vi "GeraSinalProximeter.vi"(0 "params":variant, 2 "Tx Aquisicao":dbl, 4 "estadoIn":variant) -> (15 "sinal":waveform(dbl), 18 "estadoOut":variant)   [LabVIEW 2017]
uses:
  Typedefs/Tipo_ParamsProximeter.ctl
  Typedefs/Tipo_ComponentesProximeter.ctl
  <vilib>/Analysis/NI_AALBase.lvlib
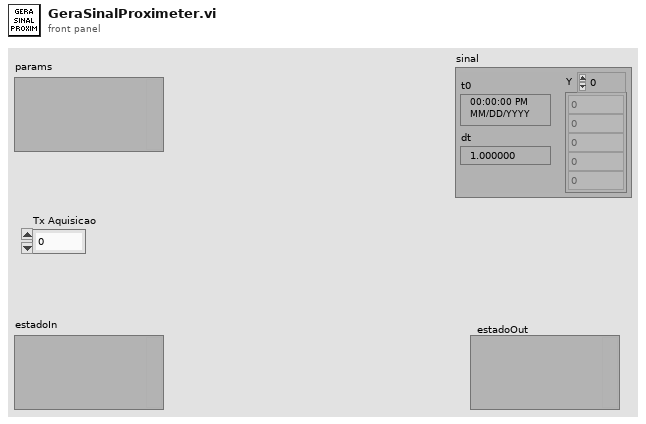
[diagram p1: front panel]
types:
  T1 = typedef "Tipo_ParamsProximeter.ctl" = cluster{"Rotacao":dbl, "Ruído":dbl, "Distância Eixo":dbl, "Fase":dbl, "Componentes":T2}
  T2 = typedef "Tipo_ComponentesProximeter.ctl" = cluster{"1xRPM":dbl, "2xRPM":dbl, "3xRPM":dbl, "4xRPM":dbl, "1/2xRPM":dbl, "1/3xRPM":dbl, "1/4xRPM":dbl, "0,45xRPM":dbl, "60Hz":dbl, "120Hz":dbl}
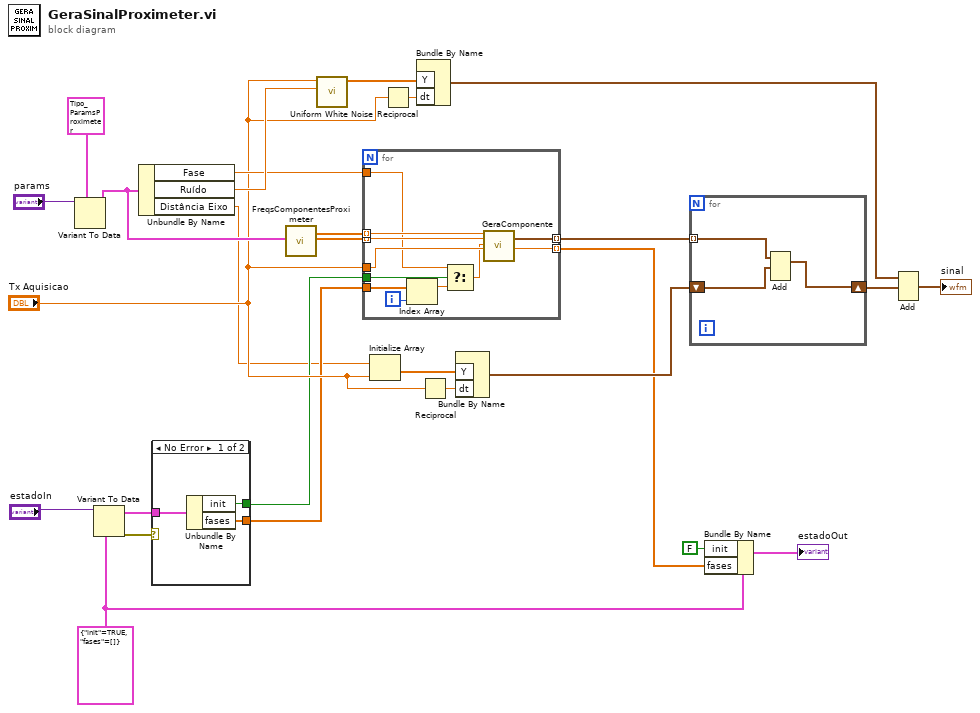
[diagram p0: block diagram]
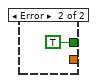
[diagram p2: hidden frame]
diagram:
  w22 = cluster{"init":bool, "fases":dbl[]} {"init"=TRUE, "fases"=[]}
  n1 = Variant To Data(type=T1 {"Rotacao"=0.0, "Ruído"=0.0, "Distância Eixo"=0.0, "Fase"=0.0, "Componentes"={"1xRPM"=0.0, "2xRPM"=0.0, "3xRPM"=0.0, "4xRPM"=0.0, "1/2xRPM"=0.0, "1/3xRPM"=0.0, "1/4xRPM"=0.0, "0,45xRPM"=0.0, "60Hz"=0.0, "120Hz"=0.0}} ("Tipo_ParamsProximeter"), Variant="params") -> (data=w10:T1)  [unwired: 1 in, 1 out]
  n2 = Variant To Data(type=w22, Variant="estadoIn") -> (data=w24:cluster{"init":bool, "fases":dbl[]}, error out=w23:errorcluster)  [unwired: 1 in]
  n3 = Unbundle By Name(w10) -> ("Fase"=w7:dbl, "Ruído"=w17:dbl, "Distância Eixo"=w1:dbl)
  n4 = case shown="No Error" w23 {
    tunnel: w24 -> [w30 _]
    tunnel: [w29 TRUE ("init")] -> w3
    tunnel: [w28 _] -> w4
    frame No Error {
      n5 = Unbundle By Name(w30) -> ("init"=w29:bool, "fases"=w28:dbl[])
    }
    frame Error {
    }
  }
  n6 = call "FreqsComponentesProximeter.vi"("Tipo_ParamsProximeter"=w10) -> ("AmplitComponentes"=w8:dbl[], "FreqsComponentes"=w9:dbl[])  [unwired: 17 in]
  n7 = call <vilib>:"Uniform White Noise.vi"("amplitude"=w17, "samples"="Tx Aquisicao") -> ("uniform white noise"=w16:dbl[])  [unwired: 8 in, 1 out]
  n8 = for {
    tunnel: w9 -> [w41] mode=indexing
    tunnel: w8 -> [w42] mode=indexing
    tunnel: w7 -> [w34]
    tunnel: "Tx Aquisicao" -> [w40]
    tunnel: [w39] -> w5 mode=indexing
    tunnel: w4 -> [w37]
    tunnel: w3 -> [w36]
    tunnel: [w32] -> w2 mode=indexing
    i -> [w38]
    n9 = Index Array(array=w37, index=w38) -> (element=w35:dbl)
    n10 = Select(t=w34, s=w36, f=w35) -> (s? t:f=w33:dbl)
    n11 = call "GeraComponente.vi"("Amplitude"=w42, "Frequencia"=w41, "Fase"=w33, "Tx Aquisicao"=w40) -> ("componente wfm"=w32:waveform(dbl), "fase saida"=w39:dbl)  [unwired: 14 in]
  }
  n12 = Initialize Array(w1, "Tx Aquisicao") -> (w13:dbl[])
  n13 = Reciprocal(x="Tx Aquisicao") -> (1/x=w15:dbl)
  n14 = Bundle By Name("Y"=w16, "dt"=w15) -> (w14:waveform(dbl))  [unwired: 1 in]
  n15 = Reciprocal(x="Tx Aquisicao") -> (1/x=w12:dbl)
  n16 = Bundle By Name("Y"=w13, "dt"=w12) -> (w11:waveform(dbl))  [unwired: 1 in]
  n17 = for {
    shift-right: [w44] -> w19
    shift-left: w11 -> [w45]
    tunnel: w2 -> [w43] mode=indexing
    n18 = Add(1:w45, 2:w43) -> (0:w44:waveform(dbl))  [unwired: 1 in, 1 out]
  }
  n19 = Bundle By Name(cluster=w22, "init"=FALSE, "fases"=w5) -> (→"estadoOut":cluster{"init":bool, "fases":dbl[]})
  n20 = Add(1:w19, 2:w14) -> (0:→"sinal":waveform(dbl))  [unwired: 1 in, 1 out]
